vi "Extreme Value Random.vi"(6 "seed":i32=-1, 7 "reset":bool, 9 "b":dbl=1.0, 10 "a":dbl, 11 "samples":i32=128) -> (0 "error":i32, 3 "extreme value random numbers":dbl[](array[numeric]))   [LabVIEW 2020, in "NI_Gmath.lvlib"]
doc: "Generates random values from a variate X, where X describes the selected distribution type. You must manually select the polymorphic instance to use."
uses:
  <vilib>/gmath/NI_Gmath.lvlib
  <vilib>/gmath/statdist.llb/st_error_code.ctl
panel:
  # "Extreme Value Random"
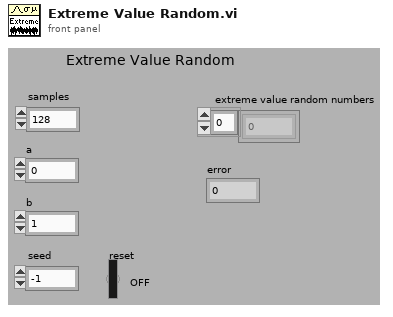
[diagram p1: front panel]
types:
  T1 = typedef "NI_Gmath.lvlib/st_error_code.ctl" = i32
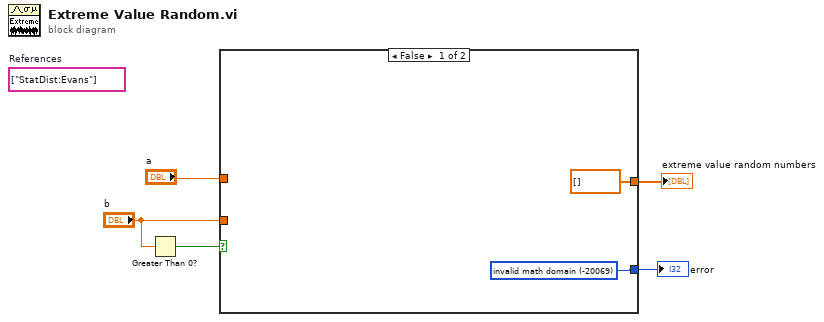
[diagram p0: block diagram]
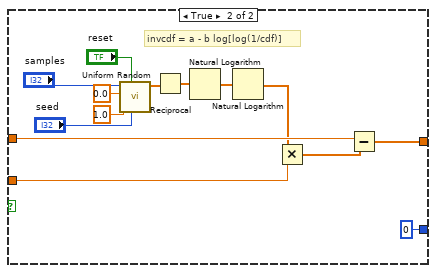
[diagram p2: hidden frame]
diagram:
  (unwired) string[] ["StatDist:Evans"]  # References
  n1 = Greater Than 0?(x="b") -> (x > 0?=w4:bool)
  n2 = case shown="False" w4 {
    tunnel: [w7 0 ("invalid math domain")] -> w2
    tunnel: [dbl[] [] w14] -> w1
    tunnel: "a" -> [_ w20]
    tunnel: "b" -> [_ w17]
    frame False {
      w7 = T1 -20069 items=["invalid math domain"=-20069, "Fourier interpolation size m >= n"=-20070, "empty array"=-20003] ("stat interp error code")
    }
    frame True {
      # "invcdf = a - b log[log(1/cdf)]"
      n3 = call <vilib>:"Uniform Random.vi"("seed"="seed", "reset"="reset", "xmax"=1.0, "xmin"=0.0, "samples"="samples") -> ("uniform random data"=w11:dbl[])  [unwired: 5 in, 1 out]
      n4 = Reciprocal(x=w11) -> (1/x=w19:dbl[])
      n5 = Natural Logarithm(1:w19) -> (0:w18:dbl[])
      n6 = Natural Logarithm(1:w18) -> (0:w16:dbl[])
      n7 = Multiply(x=w16, y=w17) -> (x*y=w15:dbl[])
      n8 = Subtract(x=w20, y=w15) -> (x-y=w14:dbl[])
    }
  }
  "error" <- w2
  "extreme value random numbers" <- w1
